vi "Andor_Initialisation.vi"(8 "error in (no error)":errorcluster) -> (0 "error out":errorcluster)   [LabVIEW 2013]
uses:
  Variables/GlobalGetCamerasOnOff.vi
  Variables/CameraStatus.vi
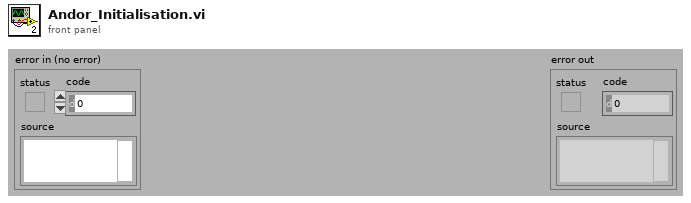
[diagram p1: front panel]
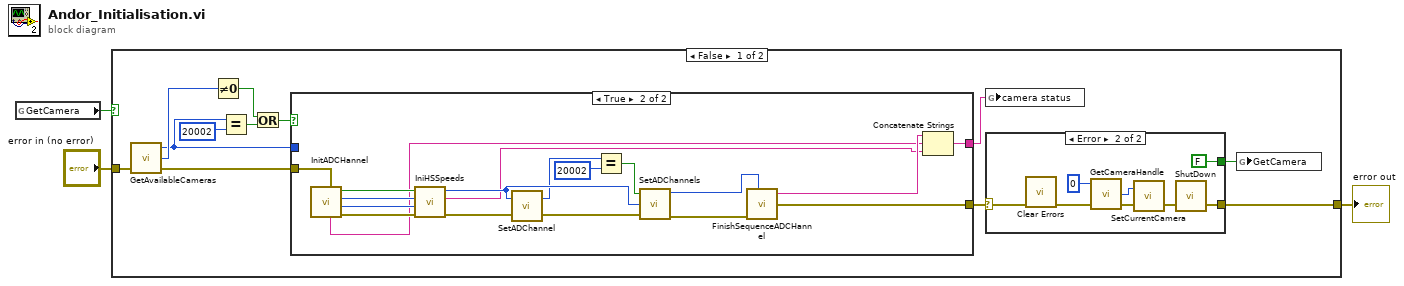
[diagram p0: block diagram]
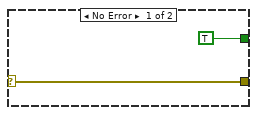
[diagram p2: hidden frame]
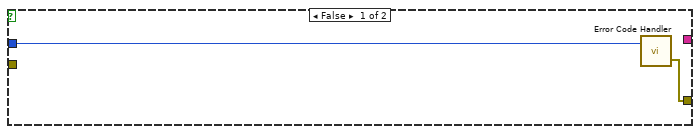
[diagram p3: hidden frame]
diagram:
  n1 = global read "GlobalGetCamerasOnOff.vi" "GetCamera"() -> (w1:bool)
  n2 = case shown="False" w1 {
    tunnel: "error in (no error)" -> [w15 w46]
    tunnel: [w8 w46] -> w2
    frame False {
      n3 = call "GetAvailableCameras.vi"("error in (no error)"=w15) -> ("error out"=w11:errorcluster, "totalCameras"=w9:i32, "DLL error code"=w6:u32)  [unwired: 2 in]
      n4 = Not Equal To 0?(x=w9) -> (x != 0?=w12:bool)
      n5 = Equal?(x=w6, y=u32 20002) -> (x = y?=w13:bool)
      n6 = Or(x=w12, y=w13) -> (x .or. y?=w10:bool)
      n7 = case shown="True" w10 {
        tunnel: w11 -> [_ w44]
        tunnel: [w27 w45] -> w5
        tunnel: w6 -> [w26 _]
        tunnel: [_ w28] -> w4
        frame False {
          n8 = call "Error Code Handler.vi"("DLL error code"=w26) -> ("error out"=w27:errorcluster)  [unwired: 1 in, 1 out]
        }
        frame True {
          n9 = call "InitADCHannel.vi"("error out"=w44) -> ("Boolean"=w43:bool, "number"=w33:i32, "DLL error code"=w32:u32, "String"=w30:string, "error out 2"=w42:errorcluster)  [unwired: 3 in]
          n10 = call "IniHSSpeeds.vi"("error out 2"=w42, "DLL error code"=w32, "number"=w33, "Boolean"=w43) -> ("error out"=w36:errorcluster, "to shell"=w29:string, "Numeric"=w35:i32)  [unwired: 1 in]
          n11 = call "SetADChannel.vi"("error in (no error)"=w36, "channel"=w35) -> ("error out"=w39:errorcluster, "DLL error code"=w34:u32)
          n12 = Equal?(x=w34, y=u32 20002) -> (x = y?=w38:bool)
          n13 = call "SetADChannels.vi"("error out"=w39, "Numeric"=w35, "Boolean"=w38) -> ("error out 2"=w41:errorcluster, "Numeric 2"=w40:i32)  [unwired: 2 in]
          n14 = call "FinishSequenceADCHannel.vi"("Numeric 2"=w40, "error out 2"=w41) -> ("to shell"=w31:string, "error out"=w45:errorcluster)  [unwired: 7 in]
          n15 = Concatenate Strings(w31, w30, w29) -> (w28:string)
        }
      }
      n16 = global write "CameraStatus.vi" "camera status"(w4) -> ()
      n17 = case shown="Error" w5 {
        selector: w5 -> [w17 w23]
        tunnel: [w17 w25] -> w8
        tunnel: [TRUE FALSE] -> w7
        frame No Error {
        }
        frame Error {
          n18 = call <vilib>:"Clear Errors.vi"("error in (no error)"=w23) -> ("error out"=w22:errorcluster)  [unwired: 6 in]
          n19 = call "GetCameraHandle.vi"("error in (no error)"=w22, "cameraIndex"=0) -> ("error out"=w21:errorcluster, "cameraHandle"=w19:i32)  [unwired: 1 in, 1 out]
          n20 = call "SetCurrentCamera.vi"("error in (no error)"=w21, "cameraHandle"=w19) -> ("error out"=w20:errorcluster)  [unwired: 1 out]
          n21 = call "ShutDown.vi"("error in (no error)"=w20) -> ("error out"=w25:errorcluster)  [unwired: 1 in, 1 out]
        }
      }
      n22 = global write "GlobalGetCamerasOnOff.vi" "GetCamera"(w7) -> ()
    }
    frame True {
    }
  }
  "error out" <- w2
